vi "WILT Populate Agilent Control.vi"(10 "Channel":string="1", 11 "Agilent1 Channels":string[][](array[string])) -> (3 "Agilent Control":T1[](array[typedef]))   [LabVIEW 2016]
uses:
  Type Definitions/WILT Agilent Channel Definition.ctl
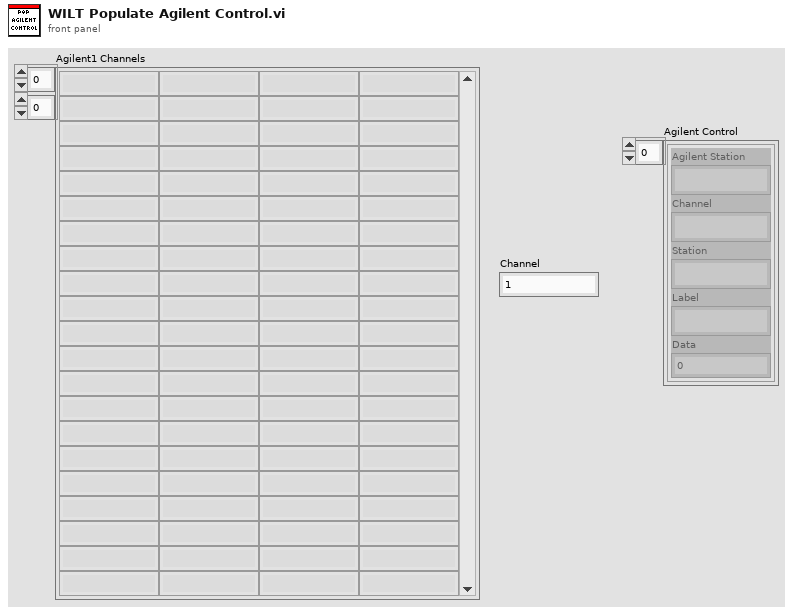
[diagram p1: front panel]
types:
  T1 = typedef "WILT Agilent Channel Definition.ctl" = cluster{"Channel":string, "Station":string, "Label":string, "Agilent Station":string, "Data":dbl}
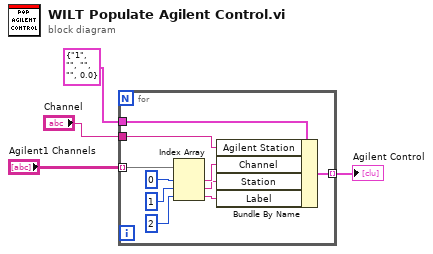
[diagram p0: block diagram]
diagram:
  n1 = for {
    tunnel: "Agilent1 Channels" -> [w12] mode=indexing
    tunnel: T1 {"Channel"="1", "Station"="", "Label"="", "Agilent Station"="", "Data"=0.0} ("Agilent Channel Definition") -> [w14]
    tunnel: [w13] -> w4 mode=indexing
    tunnel: "Channel" -> [w5]
    n2 = Index Array(array=w12, index #1=0 ("index"), index #2=1 ("index"), index #3=2 ("index")) -> (element #1=w8:string, element #2=w7:string, element #3=w6:string)
    n3 = Bundle By Name(cluster=w14, "Agilent Station"=w5, "Channel"=w8, "Station"=w7, "Label"=w6) -> (w13:T1)
  }
  "Agilent Control" <- w4
